vi "Add Definitions to Schema.vi"(8 "error in (no error)":errorcluster, 11 "JSON In":string="{}" caption="JSON Schema in") -> (0 "error out":errorcluster, 3 "JSON Out":string caption="JSON Schema out")   [LabVIEW 2023, in "JSON Schema Generator.lvlib"]
uses:
  JSON Schema Generator.lvlib
  Defintion FGV Actions.ctl
  <vilib>/JDP Science/JSONtext/Get all Object Items.vi
  <vilib>/JDP Science/JSONtext/Set Multiple Object Items.vi
  <vilib>/JDP Science/JSONtext/JSONtext.lvlib
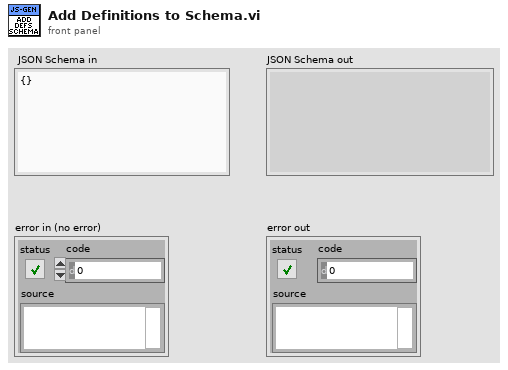
[diagram p1: front panel]
types:
  T1 = typedef "JSON Schema Generator.lvlib/Defintion FGV Actions.ctl" = enum16{"Create Defs", "Update Defs", "Get all Defs", "Get Def"}
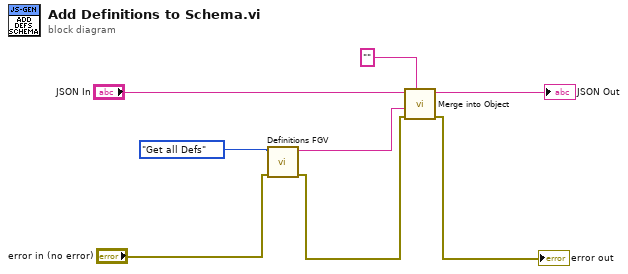
[diagram p0: block diagram]
diagram:
  n1 = call "Definitions FGV.vi"("error in (no error)"="error in (no error)", "Action"=Defintion_FGV_Actions."Get all Defs") -> ("error out"=w2:errorcluster, "Definitions out"=w4:string)  [unwired: 7 in, 1 out]
  n2 = call <vilib>:"Merge into Object.vi"("$Path or Item Name"="", "error in (no error)"=w2, "JSON Object to Merge"=w4, "JSON"="JSON In") -> ("error out"=→"error out":errorcluster, "<JSON>"=→"JSON Out":string)  [unwired: 5 in]
